vi "Calibrate Date.vi"(7 "error in":errorcluster, 10 "Instrument Handle In":i32) -> (0 "error out":errorcluster, 1 "Day":u16, 2 "Month":u16, 3 "Instrument Handle Out":i32, 4 "Year":u16)   [LabVIEW 8.6, in "ZTScopeM.lvlib"]
doc: "Query the date of the last instrument calibration."
uses:
  ZTScopeM.lvlib
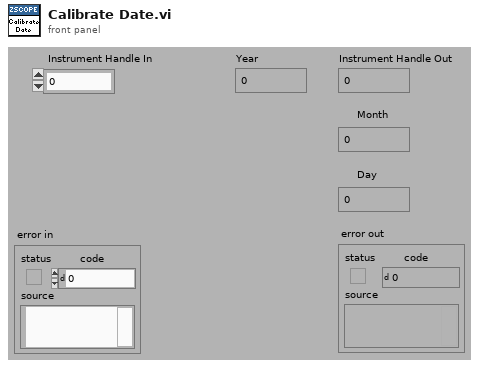
[diagram p1: front panel]
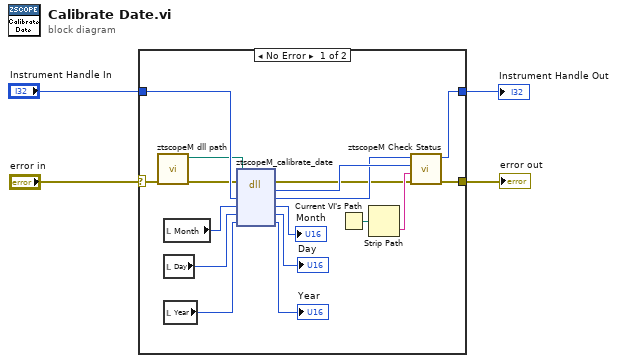
[diagram p0: block diagram]
diagram:
  n1 = case shown="No Error" "error in" {
    selector: "error in" -> [w8 w23]
    tunnel: [w13 w23] -> w1
    tunnel: "Instrument Handle In" -> [w21 w22]
    tunnel: [w14 w22] -> w3
    frame #0 {
      n2 = call "ztscopeM dll path.vi"("error in (no error)"=w8) -> ("error out"=w6:errorcluster, "<instrument>.dll path"=w7:path)  [unwired: 9 in]
      n3 = local read "Month"() -> (w20:u16)
      n4 = local read "Day"() -> (w10:u16)
      n5 = local read "Year"() -> (w9:u16)
      n6 = dll-call lib="C:/Program Files (x86)/National Instruments/LabVIEW 2013/instr.lib/ztscopem/ztscopeM.dll" fn="ztscopeM_calibrate_date"(path in=w7, error in=w6, "instrumentHandle"=w21, "Month"=w20, "Day"=w10, "Year"=w9) -> (error out=w5:errorcluster, w16:i32, "instrumentHandle"=w15:i32, "Month"=→"Month":u16, "Day"=→"Day":u16, "Year"=→"Year":u16)  [unwired: 1 in, 1 out]
      n7 = Current VI's Path() -> (path=w18:path)
      n8 = Strip Path(path=w18) -> (name=w17:string)  [unwired: 1 out]
      n9 = call "ztscopeM Check Status.vi"("error in"=w5, "name of VI"=w17, "status (return code)"=w16, "instrument handle in"=w15) -> ("error out"=w13:errorcluster, "instrument handle out"=w14:i32)  [unwired: 2 in]
    }
    frame #1 {
    }
  }
  "Instrument Handle Out" <- w3
  "error out" <- w1
